vi "CollectDataQueue.vi"(1 "ChannelArryRead":bool[](array[boolean])) -> (15 "CollectDataQueue":refnum<queue>)   [LabVIEW 2020]
uses:
  E:/01_Project/CXXXX/GKN/C18726_27program_191115004/software/DAQ/DAQ_operation_type.ctl
panel:
  out "波形图":dbl[][](graph)
  # "0手动\n1自动1阶段\n2自动2阶段"
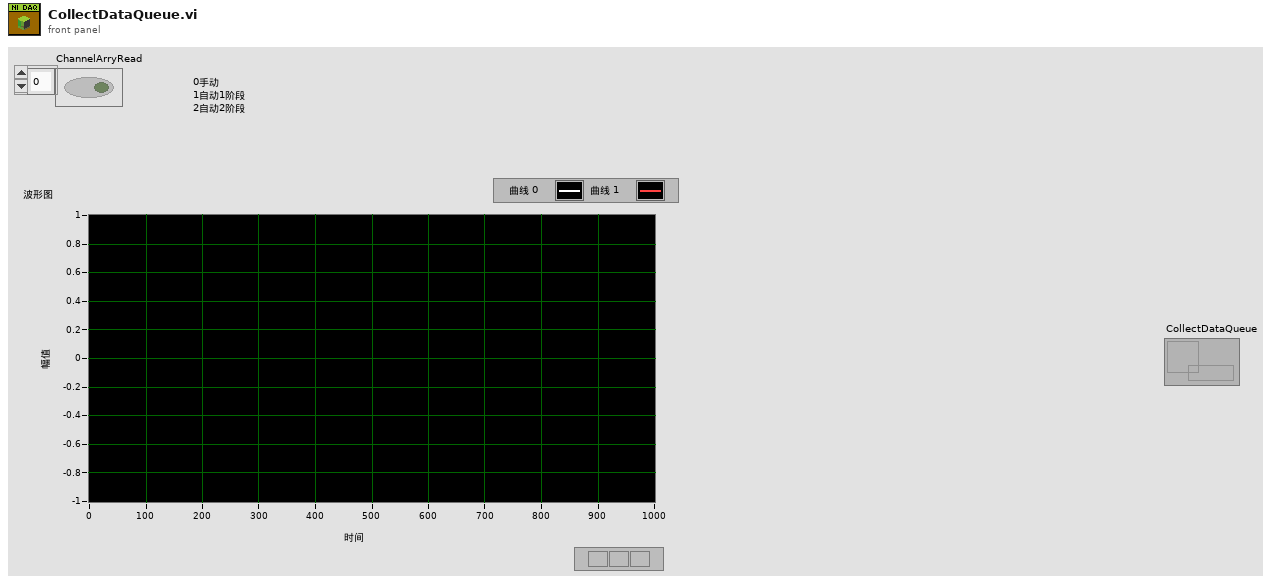
[diagram p1: front panel]
types:
  T1 = typedef "DAQ_operation_type.ctl" = enum16{"idle", "read", "write", "clear", "init", "destroy"}
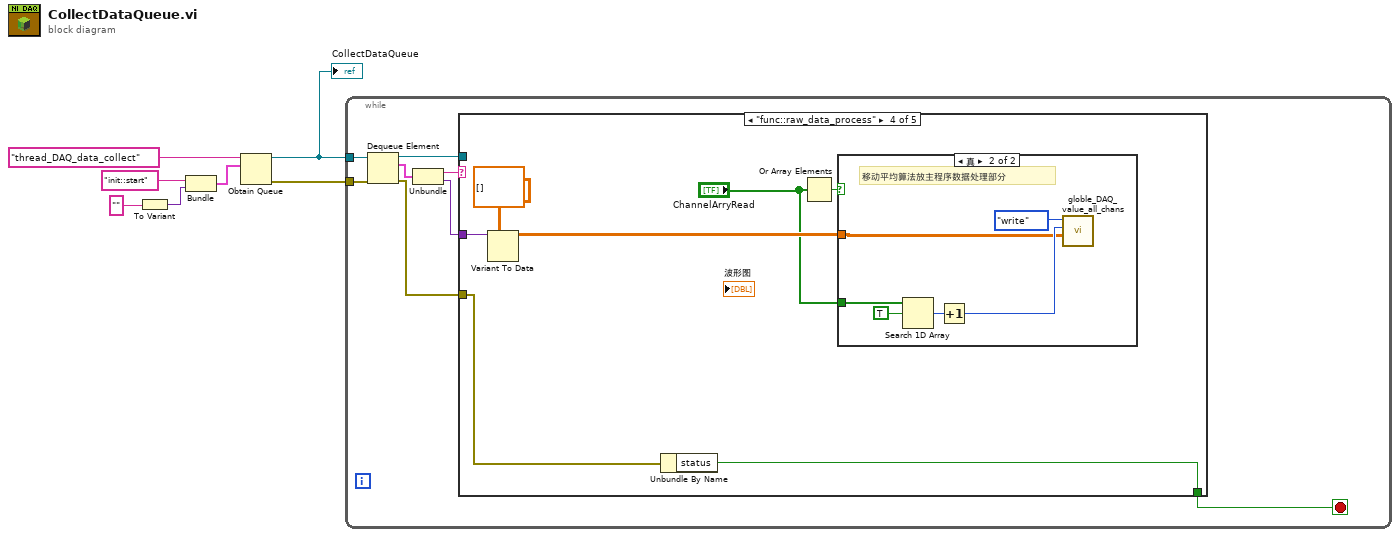
[diagram p0: block diagram]
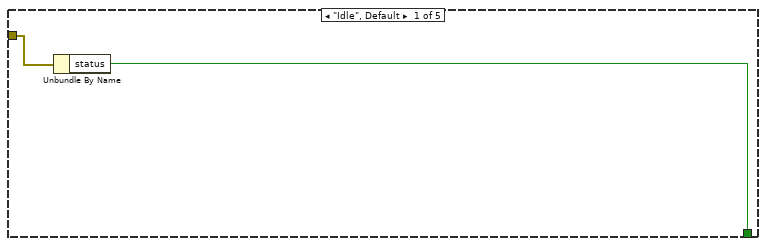
[diagram p2: hidden frame]
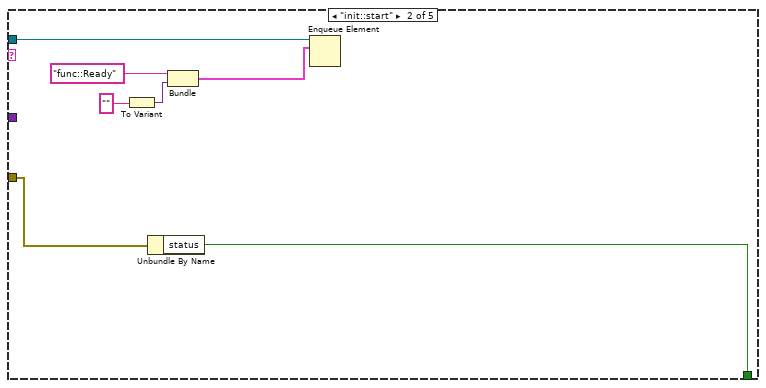
[diagram p3: hidden frame]
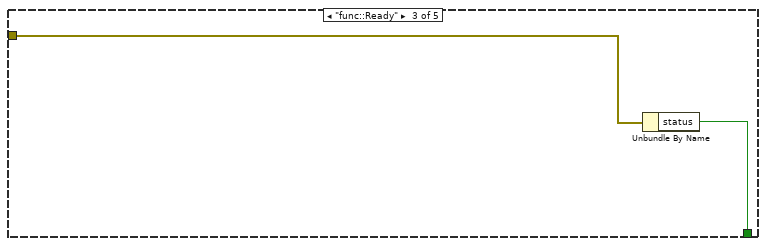
[diagram p4: hidden frame]
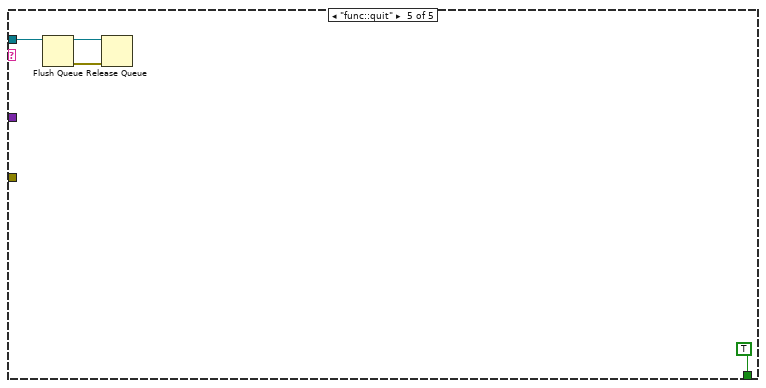
[diagram p6: hidden frame]
diagram:
  n1 = To Variant(anything="") -> (Variant=w6:variant)
  n2 = Bundle("init::start", "Variant"=w6) -> (w4:cluster{string, "Variant":variant})  [unwired: 1 in]
  n3 = Obtain Queue(name (unnamed)="thread_DAQ_data_collect" ("名称（未命名）"), element data type=w4) -> (queue out=w3:refnum<queue>, error out=w2:errorcluster)  [unwired: 3 in, 1 out]
  "CollectDataQueue" <- w3
  n4 = while {
    tunnel: w3 -> [w14]
    tunnel: w2 -> [w13]
    stop <- w9 stop-if-true
    n5 = Dequeue Element(queue=w14, error in (no error)=w13) -> (queue out=w10:refnum<queue>, element=w15:cluster{string, "Variant":variant}, error out=w8:errorcluster)  [unwired: 1 in, 1 out]
    n6 = Unbundle(w15) -> (w12:string, "Variant"=w11:variant)
    n7 = case shown="\"func::raw_data_process\"" w12 {
      tunnel: w11 -> [_ _ _ w33 _]
      tunnel: w10 -> [_ w24 _ _ w41]
      tunnel: [w16 w18 w25 w31 TRUE] -> w9
      tunnel: w8 -> [w17 w19 w26 w32 _]
      frame "Idle", Default {
        n8 = Unbundle By Name(w17) -> ("status"=w16:bool)
      }
      frame "init::start" {
        n9 = To Variant(anything="") -> (Variant=w21:variant)
        n10 = Unbundle By Name(w19) -> ("status"=w18:bool)
        n11 = Bundle("func::Ready", "Variant"=w21) -> (w20:cluster{string, "Variant":variant})  [unwired: 1 in]
        n12 = Enqueue Element(queue=w24, element=w20) -> ()  [unwired: 2 in, 3 out]
      }
      frame "func::Ready" {
        n13 = Unbundle By Name(w26) -> ("status"=w25:bool)
      }
      frame "func::raw_data_process" {
        n14 = Variant To Data(type=dbl[][] [] ("波形图"), Variant=w33) -> (data=w29:dbl[][])  [unwired: 1 in, 1 out]
        n15 = Unbundle By Name(w32) -> ("status"=w31:bool)
        n16 = Or Array Elements(Boolean array="ChannelArryRead") -> (logical OR=w28:bool)
        n17 = case shown="真" w28 {
          tunnel: w29 -> [_ w34]
          tunnel: "ChannelArryRead" -> [_ w36]
          frame False {
          }
          frame True {
            # "移动平均算法放主程序数据处理部分"
            n18 = Search 1D Array(1D array=w36, element=TRUE) -> (index of element=w37:i32)  [unwired: 1 in]
            n19 = Increment(x=w37) -> (x+1=w35:i32)
            n20 = call "globle_DAQ_value_all_chans.vi"("data_in"=w34, "chanel_nbr"=w35, "opearte"=DAQ_operation_type."write") -> ()  [unwired: 6 in, 3 out]
          }
        }
      }
      frame "func::quit" {
        n21 = Flush Queue(queue=w41) -> (queue out=w42:refnum<queue>, error out=w43:errorcluster)  [unwired: 1 in, 1 out]
        n22 = Release Queue(queue=w42, error in (no error)=w43) -> ()  [unwired: 1 in, 3 out]
      }
    }
  }
